vi "Get Images Per DMA.vi"(11 "images":u32) -> (2 "function return":u32, 3 "images out":u32)   [LabVIEW 2018, in "AndorSDK.lvlib"]
doc: "EXPNETTYPE unsigned int WINAPI GetImagesPerDMA(unsigned long * images);"
uses:
  AndorSDK.lvlib
  ATMCD32D.dll
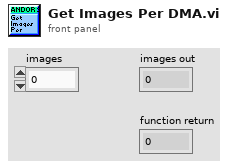
[diagram p1: front panel]
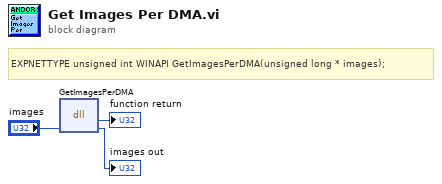
[diagram p0: block diagram]
diagram:
  # "EXPNETTYPE unsigned int WINAPI GetImagesPerDMA(unsigned long * images);"
  n1 = dll-call lib="PTH2babs E\nPersönliches02 - Arbeit03-HiwijobsLabviewCodelibANDOR\tAndor SDK\nATMCD32D.*" fn="GetImagesPerDMA"("images"="images") -> (→"function return":u32, "images"=→"images out":u32)  [unwired: 3 in, 2 out]
